vi "Clean Entry.vi"(11 "string in":string) -> (3 "string out":string)   [LabVIEW 2020]
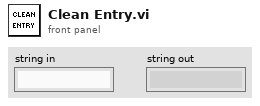
[diagram p1: front panel]
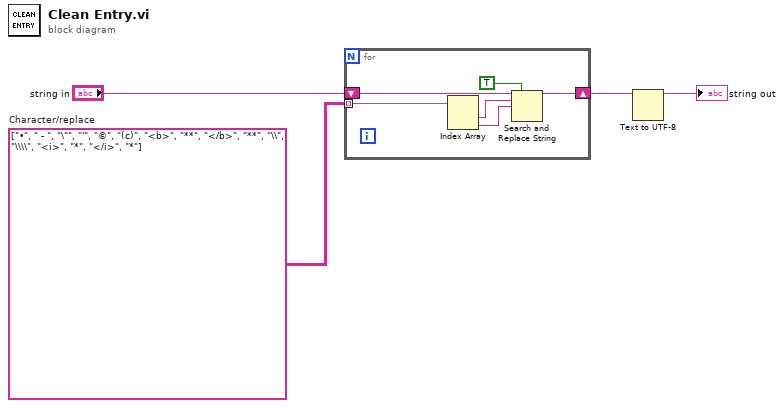
[diagram p0: block diagram]
diagram:
  w3 = string[][] [["•", " - "], ["\"", "'"], ["©", "(c)"], ["<b>", "**"], ["</b>", "**"], ["\\", "\\\\"], ["<i>", "*"], ["</i>", "*"]]  # Character/replace
  n1 = for {
    tunnel: w3 -> [w9] mode=indexing
    shift-right: [w7] -> w2
    shift-left: "string in" -> [w10]
    n2 = Index Array(array=w9) -> (element #1=w8:string, element #2=w6:string)  [unwired: 2 in]
    n3 = Search and Replace String(replace all?=TRUE, input string=w10, search string=w8, replace string=w6) -> (result string=w7:string)  [unwired: 4 in, 3 out]
  }
  n4 = Text to UTF-8(11:w2) -> (3:→"string out":string)  [unwired: 2 in, 1 out]
